vi "FFT IBN.vi"() -> ()   [LabVIEW 2016]
uses:
  RTLSDR Control/RTLSDR Global Variables.vi
  <vilib>/rvi/interface/nirviMethod/nirviMethod.xnode
  FPGA Control/FPGA Global Variables.vi
  <vilib>/rvi/interface/nirviOpenFPGA/nirviOpenFPGA.xnode
  <vilib>/FPGAPlugInAG/Dynamic/niLvFpga_Reset_Dynamic.vi
  <vilib>/FPGAPlugInAG/Dynamic/niLvFpga_Run_Dynamic.vi
  MySDR/FPGA Bitfiles/MySDRChapter3_FPGATarget_FFTIBN_+nCG0A9e09g.lvbitx
  <vilib>/FPGAPlugInAG/Dynamic/niLvFpga_ReadFifo_Dynamic.vi
  <vilib>/rvi/errors/niLvFpgaMergeErrorWithErrorCode.vi
panel:
  out "Sample Buffer":u8[](array[numeric])
  out "size(s)":i32
  out "error out":errorcluster
  out "Waveform Graph":dbl[](graph)
  in  "stop":bool
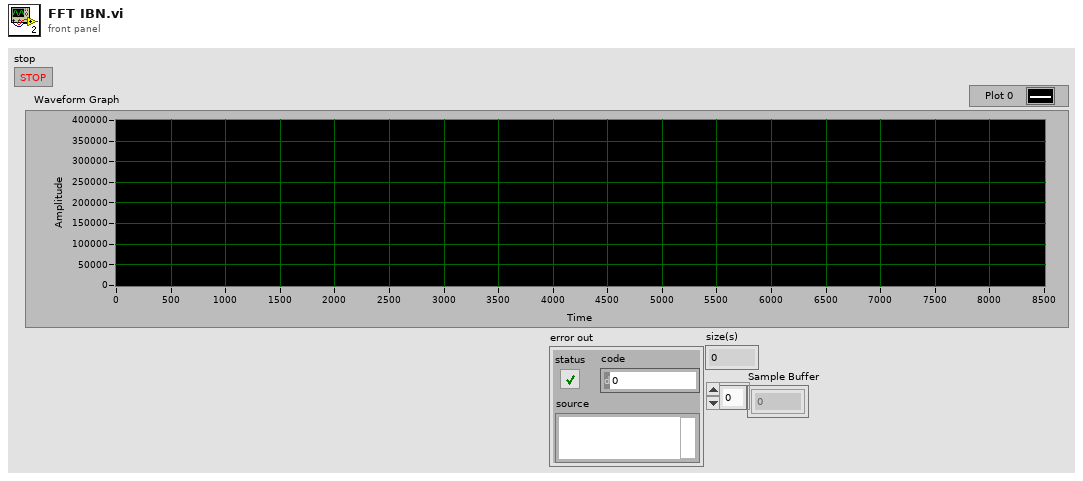
[diagram p1: front panel]
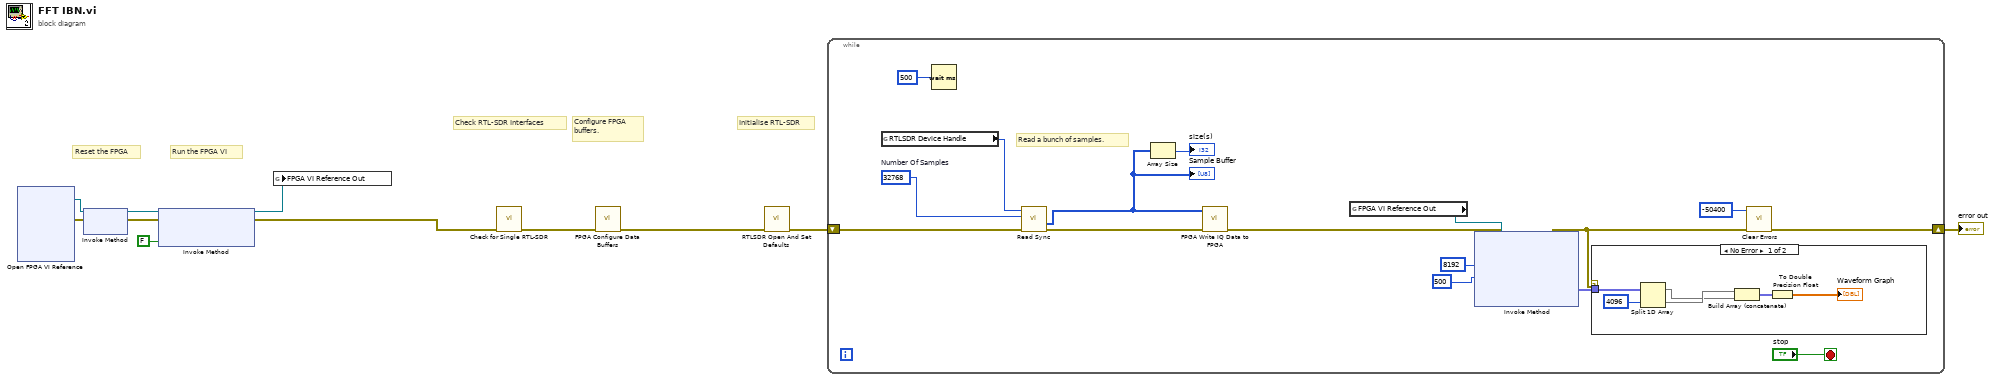
[diagram p0: block diagram]
diagram:
  # "Run the FPGA VI"
  # "Reset the FPGA"
  # "Initialise RTL-SDR"
  # "Configure FPGA\nbuffers."
  # "Check RTL-SDR Interfaces"
  n1 = xnode "Open FPGA VI Reference"() -> ("FPGA VI Reference Out"=w4:refnum<k20>, "error out"=w5:errorcluster)  [unwired: 2 in]
  n2 = xnode "Invoke Method"("FPGA VI Reference In"=w4, "error in"=w5) -> ("FPGA VI Reference Out"=w6:refnum<k20>, "error out"=w7:errorcluster)
  n3 = xnode "Invoke Method"("FPGA VI Reference In"=w6, "error in"=w7, "Wait Until Done (F)"=FALSE) -> ("FPGA VI Reference Out"=w3:refnum<k20>, "error out"=w2:errorcluster)
  n4 = global write "FPGA Global Variables.vi" "FPGA VI Reference Out"(w3) -> ()
  n5 = call "Check for Single RTL-SDR.vi"("error in (no error)"=w2) -> ("error out"=w11:errorcluster)  [unwired: 10 in]
  n6 = call "FPGA Configure Data Buffers.vi"("error in (no error)"=w11) -> ("error out"=w1:errorcluster)  [unwired: 10 in]
  n7 = call "RTLSDR Open And Set Defaults.vi"("error in (no error)"=w1) -> ("error out"=w10:errorcluster)  [unwired: 10 in]
  n8 = while {
    shift-right: [w16] -> w9
    shift-left: w10 -> [w26]
    stop <- "stop" stop-if-true
    w23 = u32 32768  # Number Of Samples
    # "Read a bunch of samples."
    n9 = global read "RTLSDR Global Variables.vi" "RTLSDR Device Handle"() -> (w27:u64)
    n10 = Wait (ms)(milliseconds to wait=u32 500) -> ()  [unwired: 1 out]
    n11 = call "Read Sync.vi"("error in (no error)"=w26, "Number Of Samples"=w23, "DeviceRefnum"=w27) -> ("error out"=w18:errorcluster, "Sample Buffer"=w14:u8[])  [unwired: 5 in, 2 out]
    "Sample Buffer" <- w14
    n12 = Array Size(array=w14) -> (size(s)=→"size(s)":i32)
    n13 = call "FPGA Write IQ Data to FPGA.vi"("error in (no error)"=w18, "Sample Buffer"=w14) -> ("error out"=w17:errorcluster)  [unwired: 9 in]
    n14 = global read "FPGA Global Variables.vi" "FPGA VI Reference Out"() -> (w22:refnum<k20>)
    n15 = xnode "Invoke Method"("FPGA VI Reference In"=w22, "error in"=w17, "Number of Elements"=u32 8192, "Timeout (ms)"=500) -> ("error out"=w12:errorcluster, "Data"=w19:fxp<+,32,24>[])  [unwired: 2 out]
    n16 = case shown="No Error" w12 {
      tunnel: w19 -> [w30 _]
      frame No Error {
        n17 = Split 1D Array(array=w30, index=4096) -> (first subarray=w29:fxp<+,32,24>[], second subarray=w32:fxp<+,32,24>[])
        n18 = Build Array (concatenate)(w32, w29) -> (w33:fxp<+,32,24>[])
        n19 = To Double Precision Float(number=w33) -> (double precision float=→"Waveform Graph":dbl[])
      }
      frame Error {
      }
    }
    n20 = call <vilib>:"Clear Errors.vi"("error in (no error)"=w12, "specific error code to clear (0: all)"=-50400) -> ("error out"=w16:errorcluster)  [unwired: 4 in, 1 out]
  }
  "error out" <- w9
